vi "VI.Launch.vi"(8 "error in (no error)":errorcluster, 11 "state variables in":T4) -> (0 "error out":errorcluster, 3 "state variables out":T4)   [LabVIEW 2015, in "Multihead GUI.lvlib"]
uses:
  Multihead GUI.lvlib
  <vilib>/NI Veristand/Execution/Workspace/WorkspaceAPI.ctl
  NationalInstruments.VeriStand.ClientAPI
  <vilib>/NI Veristand/Execution/Workspace/SystemStateEventRef.ctl
  <vilib>/NI Veristand/Execution/Workspace/Target State Info.ctl
  <vilib>/NI Veristand/Execution/Workspace/Target State.ctl
  <vilib>/NI Veristand/Execution/Workspace/SystemStateRegEventRef.ctl
  <vilib>/picture/picture.llb/imagedata.ctl
  Execution GUI/Single Station Execution.lvlib
  Overview GUI/Overview GUI.lvlib
  <vilib>/NI Veristand/Execution/Workspace/NI_VS Workspace ExecutionAPI.lvlib
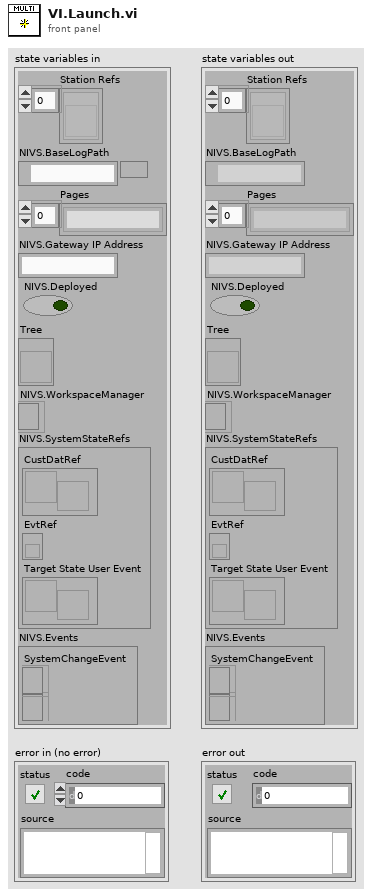
[diagram p1: front panel]
types:
  T1 = typedef "NI_VS Workspace ExecutionAPI.lvlib/WorkspaceAPI.ctl" = refnum<k24>
  T2 = typedef "NI_VS Workspace ExecutionAPI.lvlib/SystemStateEventRef.ctl" = cluster{"CustDatRef":refnum<user-event>, "EvtRef":refnum<k27>, "Target State User Event":refnum<user-event>}
  T3 = typedef "NI_VS Workspace ExecutionAPI.lvlib/SystemStateRegEventRef.ctl" = refnum<event-registration>
  T4 = cluster{"Station Refs":refnum<vi>[], "NIVS.BaseLogPath":path, "Pages":string[], "NIVS.Gateway IP Address":string, "NIVS.Deployed":bool, "Tree":refnum<vi>, "NIVS.WorkspaceManager":T1, "NIVS.SystemStateRefs":T2, "NIVS.Events":cluster{"SystemChangeEvent":T3, "WorkspaceEvent":refnum<event-registration>}}
  T5 = typedef "imagedata.ctl" = cluster{"image type":i32, "image depth":i32, "image":u8[], "mask":u8[], "colors":u32[], "Rectangle":cluster{"left":i16, "top":i16, "right":i16, "bottom":i16}}
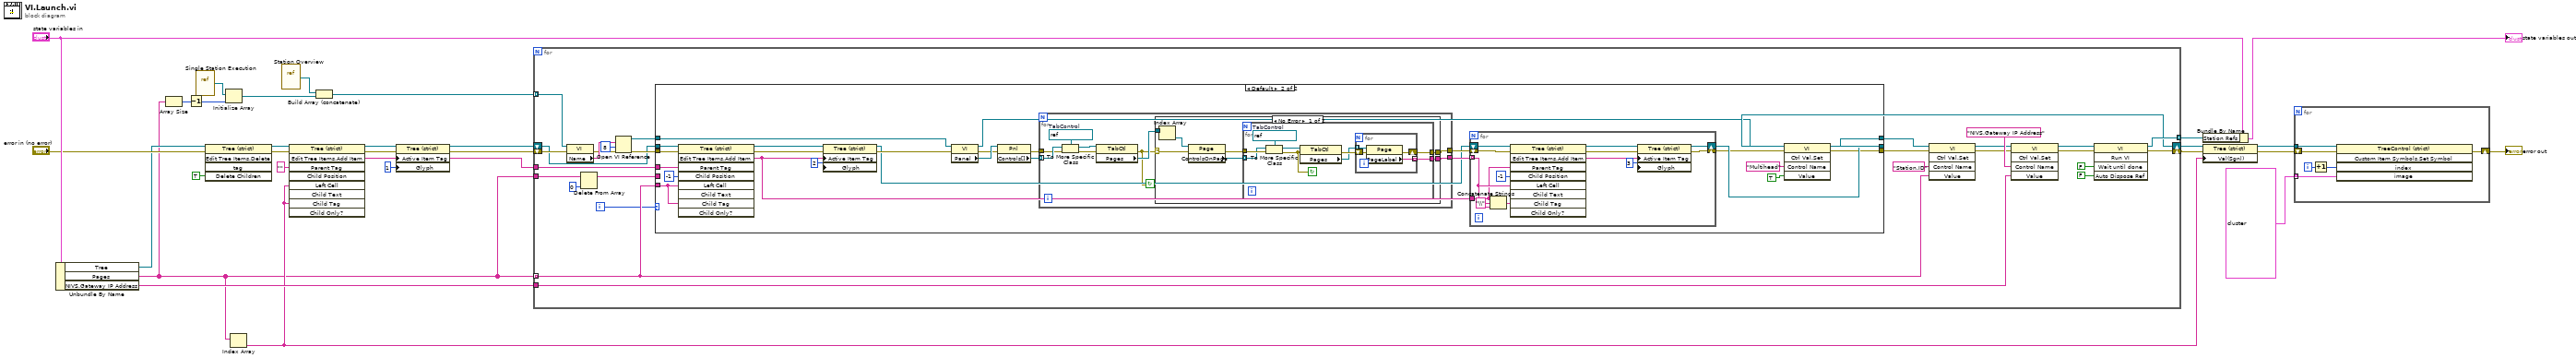
[diagram p0: block diagram]
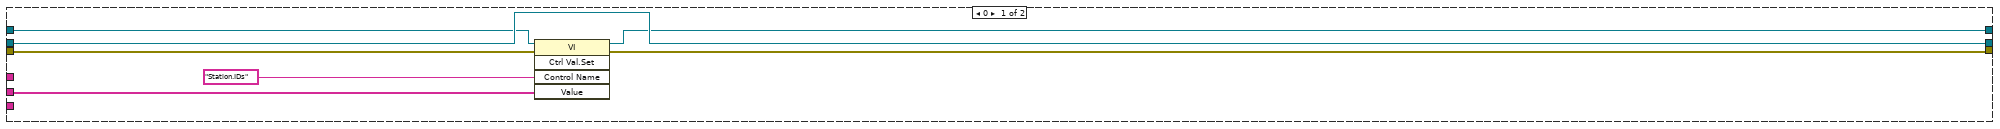
[diagram p2: hidden frame]
diagram:
  n1 = Unbundle By Name("state variables in") -> ("Tree"=w17:refnum<vi>, "Pages"=w1:string[], "NIVS.Gateway IP Address"=w30:string)
  n2 = Array Size(array=w1) -> (size(s)=w6:i32)
  n3 = Decrement(x=w6) -> (x-1=w5:i32)
  n4 = vi-ref "Single Station Execution.vi"() -> (w3:refnum<vi>)
  n5 = invoke class="Tree (strict)" method="Edit Tree Items.Delete"(reference=w17, error in="error in (no error)", "Delete Children"=TRUE ("Delete Children?")) -> (reference out=w20:refnum<vi>, error out=w21:errorcluster)  [unwired: 2 in, 3 out]
  n6 = Initialize Array(w3, w5) -> (w4:refnum<vi>[])
  n7 = Index Array(array=w1) -> (element=w2:string)  [unwired: 1 in]
  n8 = vi-ref "Station Overview.vi"() -> (w28:refnum<vi>)
  n9 = invoke class="Tree (strict)" method="Edit Tree Items.Add Item"(reference=w20, error in=w21, "Parent Tag"="", "Left Cell"=w2, "Child Tag"=w2) -> (reference out=w8:refnum<vi>, error out=w15:errorcluster, "Edit Tree Items:Add Item"=w16:string)  [unwired: 4 in, 6 out]
  n10 = Build Array (concatenate)(w28, w4) -> (w25:refnum<vi>[])
  n11 = property class="Tree (strict)"(reference=w8, error in=w15, "Active Item Tag"=w16, "Glyph"=1 ("Active Item:Symbol Index")) -> (reference out=w7:refnum<vi>, error out=w14:errorcluster)
  n12 = for {
    tunnel: w25 -> [w58] mode=indexing
    shift-right: [w55] -> w24
    shift-left: w14 -> [w39]
    tunnel: [w53] -> w26 mode=indexing
    tunnel: w1 -> [w42] mode=indexing
    tunnel: w30 -> [w46]
    tunnel: w1 -> [w45]
    tunnel: w16 -> [w43]
    shift-right: [w36] -> w18
    shift-left: w7 -> [w38]
    i -> [w37]
    n13 = property class="VI"(reference=w58, error in=w39) -> (error out=w54:errorcluster, "Name"=w57:string)  [unwired: 1 out]
    n14 = Delete From Array(array=w45, index=0) -> (array with subset deleted=w35:string[])  [unwired: 1 in, 1 out]
    n15 = Open VI Reference(vi path=w57, options=8, error in (no error)=w54) -> (vi reference=w40:refnum<vi>, error out=w41:errorcluster)  [unwired: 3 in]
    n16 = case shown="Default" w37 {
      tunnel: w43 -> [_ w90]
      tunnel: w42 -> [_ w89]
      tunnel: w41 -> [w63 w82]
      tunnel: w40 -> [w61 w81]
      tunnel: [w60 w73] -> w33
      tunnel: [w62 w75] -> w34
      tunnel: w38 -> [w65 w80]
      tunnel: [w65 w79] -> w36
      tunnel: w35 -> [w59 _]
      frame 0 {
        n17 = invoke class="VI" method="Ctrl Val.Set"(reference=w61, error in=w63, "Control Name"="Station.IDs", "Value"=w59) -> (reference out=w60:refnum<vi>, error out=w62:errorcluster)  [unwired: 1 in, 3 out]
      }
      frame Default {
        n18 = invoke class="Tree (strict)" method="Edit Tree Items.Add Item"(reference=w80, error in=w82, "Parent Tag"=w90, "Child Position"=-1, "Left Cell"=w89, "Child Tag"=w89) -> (reference out=w67:refnum<vi>, error out=w69:errorcluster, "Edit Tree Items:Add Item"=w70:string)  [unwired: 3 in, 6 out]
        n19 = property class="Tree (strict)"(reference=w67, error in=w69, "Active Item Tag"=w70, "Glyph"=2 ("Active Item:Symbol Index")) -> (reference out=w66:refnum<vi>, error out=w68:errorcluster)
        n20 = property class="VI"(reference=w81, error in=w68) -> (reference out=w74:refnum<vi>, error out=w86:errorcluster, "Panel"=w88:refnum<vi>)
        n21 = property class="Pnl"(reference=w88, error in=w86) -> (error out=w85:errorcluster, "Controls[]"=w87:refnum<vi>[])  [unwired: 1 out]
        n22 = for {
          tunnel: w87 -> [w112] mode=indexing
          tunnel: w85 -> [w110]
          tunnel: [w106] -> w84
          tunnel: [w105] -> w83
          stop <- w104 continue-if-true
          w111 = refnum<vi> refnum  # TabControl
          n23 = To More Specific Class(target class=w111, reference=w112, error in=w110) -> (specific class reference=w109:refnum<vi>, error out=w108:errorcluster)
          n24 = property class="TabCtl"(reference=w109, error in=w108) -> (error out=w104:errorcluster, "Pages"=w107:refnum<vi>[])  [unwired: 1 out]
          n25 = case shown="No Error" w104 {
            selector: w104 -> [w113 w133]
            tunnel: w107 -> [w119 _]
            tunnel: [w115 _] -> w106
            tunnel: [w114 w133] -> w105
            frame No Error {
              n26 = Index Array(array=w119) -> (element=w118:refnum<vi>)  [unwired: 1 in]
              n27 = property class="Page"(reference=w118, error in=w113) -> (error out=w117:errorcluster, "ControlsOnPage"=w116:refnum<vi>[])  [unwired: 1 out]
              n28 = for {
                tunnel: [w126] -> w115
                tunnel: [w125] -> w114
                tunnel: w117 -> [w121]
                tunnel: w116 -> [w120] mode=indexing
                stop <- w122 continue-if-true
                w128 = refnum<vi> refnum  # TabControl
                n29 = To More Specific Class(target class=w128, reference=w120, error in=w121) -> (specific class reference=w127:refnum<vi>, error out=w122:errorcluster)
                n30 = property class="TabCtl"(reference=w127, error in=w122) -> (error out=w124:errorcluster, "Pages"=w123:refnum<vi>[])  [unwired: 1 out]
                n31 = for {
                  tunnel: w123 -> [w131] mode=indexing
                  tunnel: [w130] -> w126 mode=indexing
                  shift-right: [w129] -> w125
                  shift-left: w124 -> [w132]
                  n32 = property class="Page"(reference=w131, error in=w132) -> (error out=w129:errorcluster, "PageLabel"=w130:string)  [unwired: 1 out]
                }
              }
            }
            frame Error {
            }
          }
        }
        n33 = for {
          tunnel: w84 -> [w102] mode=indexing
          shift-right: [w92] -> w76
          shift-left: w83 -> [w103]
          tunnel: w70 -> [w98]
          shift-right: [w91] -> w79
          shift-left: w66 -> [w99]
          n34 = Concatenate Strings(w98, "\\" ("string"), w102) -> (w101:string)
          n35 = invoke class="Tree (strict)" method="Edit Tree Items.Add Item"(reference=w99, error in=w103, "Parent Tag"=w98, "Child Position"=-1, "Left Cell"=w102, "Child Tag"=w101) -> (reference out=w94:refnum<vi>, error out=w93:errorcluster, "Edit Tree Items:Add Item"=w95:string)  [unwired: 3 in, 6 out]
          n36 = property class="Tree (strict)"(reference=w94, error in=w93, "Active Item Tag"=w95, "Glyph"=3 ("Active Item:Symbol Index")) -> (reference out=w91:refnum<vi>, error out=w92:errorcluster)
        }
        n37 = invoke class="VI" method="Ctrl Val.Set"(reference=w74, error in=w76, "Control Name"="Multihead", "Value"=TRUE) -> (reference out=w73:refnum<vi>, error out=w75:errorcluster)  [unwired: 1 in, 3 out]
      }
    }
    n38 = invoke class="VI" method="Ctrl Val.Set"(reference=w33, error in=w34, "Control Name"="Station.ID", "Value"=w42) -> (reference out=w31:refnum<vi>, error out=w32:errorcluster)  [unwired: 1 in, 3 out]
    n39 = invoke class="VI" method="Ctrl Val.Set"(reference=w31, error in=w32, "Control Name"="NIVS.Gateway IP Address", "Value"=w46) -> (reference out=w49:refnum<vi>, error out=w48:errorcluster)  [unwired: 1 in, 3 out]
    n40 = invoke class="VI" method="Run VI"(reference=w49, error in=w48, "Wait until done"=FALSE ("Wait Until Done"), "Auto Dispose Ref"=FALSE ("Auto Dispose Reference")) -> (reference out=w53:refnum<vi>, error out=w55:errorcluster)  [unwired: 1 in, 3 out]
  }
  n41 = Bundle By Name(cluster="state variables in", "Station Refs"=w26) -> (→"state variables out":T4)
  n42 = property class="Tree (strict)"(reference=w18, error in=w24, "Val(Sgnl)"=w2) -> (reference out=w11:refnum<vi>, error out=w10:errorcluster)
  n43 = for {
    tunnel: T5[] [{"image type"=0, "image depth"=32, "image"=array[1024 elements], "mask"=[14, 0, 63, 128, 255, 224, 255, 240, 255, 240, 255, 240, 255, 248, 127, 254, 63, 255, 15, 255, 15, 255, 15, 255, 7, 255, 3, 255, 0, 254, 0, 56], "colors"=[], "Rectangle"={"left"=0, "top"=0, "right"=16, "bottom"=16}}, {"image type"=0, "image depth"=24, "image"=[255, 255, 255, 255, 255, 255, 255, 255, 255, 255, 255, 255, 255, 255, 255, 255, 255, 255, 0, 0, 255, 0, 0, 255, 255, 255, 255, 255, 0, 0, 255, 0, 0, 192, 192, 192, 255, 255, 255, 255, 255, 255, 255, 0, 0, 255, 0, 0, 255, 255, 255, 255, 255, 255, 255, 255, 255, 255, 255, 255, 255, 255, 255, 0, 0, 255, 0, 0, 255, 0, 0, 255, 255, 255, 255, 255, 0, 0, 255, 0, 0, 255, 0, 0, 192, 192, 192, 255, 0, 0, 255, 0, 0, 255, 0, 0, 255, 255, 255, 255, 255, 255, 255, 255, 255, 255, 255, 255, 0, 0, 255, 0, 0, 255, 0, 0, 255, 192, 192, 192, 255, 255, 255, 255, 255, 255, 255, 0, 0, 255, 0, 0, 255, 0, 0, 255, 0, 0, 255, 0, 0, 192, 192, 192, 0, 0, 255, 0, 0, 255, 255, 255, 255, 0, 0, 255, 0, 0, 255, 0, 0, 255, 192, 192, 192, 255, 255, 255, 255, 255, 255, 255, 255, 255, 255, 255, 255, 255, 0, 0, 255, 0, 0, 255, 0, 0, 192, 192, 192, 255, 255, 255, 0, 0, 255, 0, 0, 255, 0, 0, 255, 0, 0, 255, 0, 0, 255, 192, 192, 192, 255, 255, 255, 255, 255, 255, 255, 255, 255, 255, 255, 255, 255, 0, 0, 255, 0, 0, 255, 0, 0, 255, 0, 0, 255, 0, 0, 192, 192, 192, 255, 255, 255, 0, 0, 255, 0, 0, 255, 0, 0, 255, 192, 192, 192, 255, 255, 255, 255, 255, 255, 255, 255, 255, 255, 255, 255, 255, 0, 0, 255, 0, 0, 255, 0, 0, 192, 192, 192, 255, 0, 0, 255, 0, 0, 255, 0, 0, 255, 255, 255, 255, 255, 255, 0, 0, 255, 192, 192, 192, 255, 255, 255, 255, 255, 255, 255, 255, 255, 255, 255, 255, 255, 255, 255, 255, 0, 0, 255, 0, 0, 192, 192, 192, 255, 255, 253, 255, 255, 253, 255, 0, 0, 255, 0, 0, 255, 255, 255, 255, 255, 255, 255, 255, 255, 255, 255, 255, 0, 128, 0, 0, 128, 0, 0, 128, 0, 0, 128, 0, 0, 128, 0, 0, 128, 0, 0, 128, 0, 0, 128, 0, 0, 128, 0, 0, 0, 0, 255, 255, 255, 255, 255, 255, 255, 255, 255, 255, 255, 255, 255, 255, 255, 255, 255, 255, 0, 128, 0, 0, 128, 0, 0, 128, 0, 0, 0, 0, 255, 255, 253, 0, 128, 0, 255, 255, 253, 0, 0, 0, 0, 128, 0, 0, 0, 0, 255, 255, 255, 255, 255, 255, 255, 255, 255, 255, 255, 255, 255, 255, 255, 255, 255, 255, 0, 128, 0, 0, 128, 0, 0, 128, 0, 0, 128, 0, 0, 128, 0, 0, 128, 0, 0, 128, 0, 0, 128, 0, 0, 128, 0, 0, 0, 0, 255, 255, 255, 255, 255, 255, 255, 255, 255, 255, 255, 255, 255, 255, 255, 255, 255, 255, 0, 128, 0, 0, 0, 0, 255, 255, 253, 0, 128, 0, 0, 128, 0, 0, 0, 0, 255, 255, 253, 0, 128, 0, 0, 128, 0, 0, 0, 0, 255, 255, 255, 255, 255, 255, 255, 255, 255, 255, 255, 255, 255, 255, 255, 255, 255, 255, 0, 128, 0, 0, 128, 0, 0, 128, 0, 0, 128, 0, 0, 128, 0, 0, 128, 0, 0, 128, 0, 0, 128, 0, 0, 128, 0, 0, 0, 0, 255, 255, 255, 255, 255, 255, 255, 255, 255, 255, 255, 255, 255, 255, 255, 255, 255, 255, 0, 0, 0, 0, 0, 0, 0, 0, 0, 0, 0, 0, 0, 0, 0, 0, 0, 0, 0, 0, 0, 0, 0, 0, 0, 0, 0, 0, 0, 0, 255, 255, 255, 255, 255, 255], "mask"=[], "colors"=[], "Rectangle"={"left"=0, "top"=0, "right"=16, "bottom"=13}}, {"image type"=0, "image depth"=24, "image"=[0, 0, 0, 0, 0, 0, 0, 0, 0, 0, 0, 0, 0, 0, 0, 0, 0, 0, 0, 0, 0, 0, 0, 0, 0, 0, 0, 0, 0, 0, 0, 0, 0, 0, 0, 0, 0, 0, 0, 0, 0, 0, 255, 255, 255, 255, 255, 255, 0, 0, 0, 0, 153, 255, 0, 153, 255, 0, 153, 255, 0, 153, 255, 0, 153, 255, 0, 153, 255, 0, 153, 255, 0, 153, 255, 0, 153, 255, 0, 153, 255, 0, 153, 255, 0, 153, 255, 0, 0, 0, 255, 255, 255, 255, 255, 255, 0, 0, 0, 0, 0, 0, 0, 0, 0, 0, 0, 0, 0, 0, 0, 0, 0, 0, 0, 0, 0, 0, 0, 0, 0, 0, 0, 0, 0, 0, 0, 0, 0, 0, 0, 0, 0, 0, 0, 0, 0, 0, 255, 255, 255, 255, 255, 255, 0, 0, 0, 221, 221, 221, 221, 221, 221, 221, 221, 221, 221, 221, 221, 221, 221, 221, 221, 221, 221, 221, 221, 221, 221, 221, 221, 221, 221, 221, 221, 221, 221, 221, 221, 221, 221, 221, 221, 0, 0, 0, 255, 255, 255, 255, 255, 255, 0, 0, 0, 221, 221, 221, 221, 221, 221, 221, 221, 221, 221, 221, 221, 221, 221, 221, 221, 221, 221, 221, 221, 221, 221, 221, 221, 221, 221, 221, 221, 221, 221, 221, 221, 221, 221, 221, 221, 0, 0, 0, 255, 255, 255, 255, 255, 255, 0, 0, 0, 221, 221, 221, 221, 221, 221, 119, 119, 119, 119, 119, 119, 119, 119, 119, 0, 0, 0, 221, 221, 221, 119, 119, 119, 119, 119, 119, 119, 119, 119, 0, 0, 0, 221, 221, 221, 0, 0, 0, 255, 255, 255, 255, 255, 255, 0, 0, 0, 221, 221, 221, 221, 221, 221, 119, 119, 119, 221, 221, 221, 221, 221, 221, 0, 0, 0, 221, 221, 221, 119, 119, 119, 221, 221, 221, 221, 221, 221, 0, 0, 0, 221, 221, 221, 0, 0, 0, 255, 255, 255, 255, 255, 255, 0, 0, 0, 221, 221, 221, 221, 221, 221, 0, 0, 0, 0, 0, 0, 0, 0, 0, 0, 0, 0, 221, 221, 221, 0, 0, 0, 0, 0, 0, 0, 0, 0, 0, 0, 0, 221, 221, 221, 0, 0, 0, 255, 255, 255, 255, 255, 255, 0, 0, 0, 221, 221, 221, 221, 221, 221, 221, 221, 221, 221, 221, 221, 221, 221, 221, 221, 221, 221, 221, 221, 221, 221, 221, 221, 221, 221, 221, 221, 221, 221, 221, 221, 221, 221, 221, 221, 0, 0, 0, 255, 255, 255, 255, 255, 255, 0, 0, 0, 221, 221, 221, 221, 221, 221, 221, 221, 221, 221, 221, 221, 221, 221, 221, 221, 221, 221, 221, 221, 221, 119, 119, 119, 119, 119, 119, 119, 119, 119, 0, 0, 0, 221, 221, 221, 0, 0, 0, 255, 255, 255, 255, 255, 255, 0, 0, 0, 221, 221, 221, 221, 221, 221, 221, 221, 221, 221, 221, 221, 221, 221, 221, 221, 221, 221, 221, 221, 221, 119, 119, 119, 221, 221, 221, 221, 221, 221, 0, 0, 0, 221, 221, 221, 0, 0, 0, 255, 255, 255, 255, 255, 255, 0, 0, 0, 221, 221, 221, 221, 221, 221, 221, 221, 221, 221, 221, 221, 221, 221, 221, 221, 221, 221, 221, 221, 221, 0, 0, 0, 0, 0, 0, 0, 0, 0, 0, 0, 0, 221, 221, 221, 0, 0, 0, 255, 255, 255, 255, 255, 255, 0, 0, 0, 221, 221, 221, 221, 221, 221, 221, 221, 221, 221, 221, 221, 221, 221, 221, 221, 221, 221, 221, 221, 221, 221, 221, 221, 221, 221, 221, 221, 221, 221, 221, 221, 221, 221, 221, 221, 0, 0, 0, 255, 255, 255, 255, 255, 255, 0, 0, 0, 221, 221, 221, 221, 221, 221, 221, 221, 221, 221, 221, 221, 221, 221, 221, 221, 221, 221, 221, 221, 221, 221, 221, 221, 221, 221, 221, 221, 221, 221, 221, 221, 221, 221, 221, 221, 0, 0, 0, 255, 255, 255, 255, 255, 255, 0, 0, 0, 0, 0, 0, 0, 0, 0, 0, 0, 0, 0, 0, 0, 0, 0, 0, 0, 0, 0, 0, 0, 0, 0, 0, 0, 0, 0, 0, 0, 0, 0, 0, 0, 0, 0, 0, 0, 0, 0, 0, 255, 255, 255, 255, 255, 255, 255, 255, 255, 255, 255, 255, 255, 255, 255, 255, 255, 255, 255, 255, 255, 255, 255, 255, 255, 255, 255, 255, 255, 255, 255, 255, 255, 255, 255, 255, 255, 255, 255, 255, 255, 255, 255, 255, 255, 255, 255, 255, 255, 255, 255, 255, 255, 255], "mask"=[], "colors"=[], "Rectangle"={"left"=0, "top"=0, "right"=16, "bottom"=16}}] ("Array") -> [w139] mode=indexing
    tunnel: w11 -> [w137]
    shift-right: [w135] -> w9
    shift-left: w10 -> [w136]
    i -> [w138]
    n44 = Increment(x=w138) -> (x+1=w134:i32)
    n45 = invoke on="Invoke Node" class="TreeControl (strict)" method="Custom Item Symbols.Set Symbol"(reference=w137, error in=w136, "index"=w134, "image"=w139) -> (error out=w135:errorcluster)  [unwired: 1 in, 4 out]
  }
  "error out" <- w9
